vi "Test Gain.vi"(8 "error in (no error)":errorcluster, 11 "Instrument.Lockin in":refnum<class "Instrument.Lockin.lvclass">) -> (0 "error out":errorcluster, 3 "Instrument.Lockin out":refnum<class "Instrument.Lockin.lvclass">)   [LabVIEW 2019]
uses:
  src/Instrument.Lockin/Instrument.Lockin.lvclass
  <vilib>/addons/_JKI Toolkits/Caraya/classes/Assert/Assert Equal Value_Variant.vi
  <vilib>/addons/_JKI Toolkits/Caraya/classes/Test/Test.lvclass
  <vilib>/addons/_JKI Toolkits/Caraya/classes/Assert/Assert.lvclass
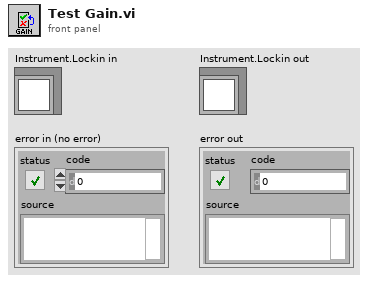
[diagram p1: front panel]
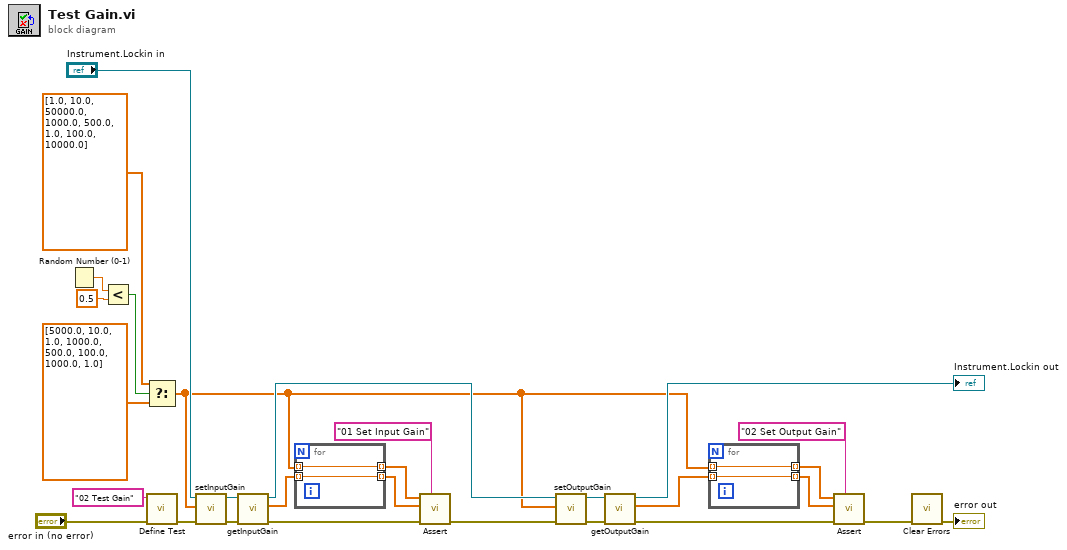
[diagram p0: block diagram]
diagram:
  n1 = Random Number (0-1)() -> (number: 0 to 1=w24:dbl)
  n2 = Less?(x=w24, y=0.5) -> (x < y?=w21:bool)
  n3 = Select(t=dbl[] [1.0, 10.0, 50000.0, 1000.0, 500.0, 1.0, 100.0, 10000.0] ("Gain"), s=w21, f=dbl[] [5000.0, 10.0, 1.0, 1000.0, 500.0, 100.0, 1000.0, 1.0] ("Gain")) -> (s? t:f=w1:dbl[])
  n4 = call <vilib>:"Define Test.vi"("error in (no error)"="error in (no error)", "Label (VI Title)"="02 Test Gain") -> ("error out"=w29:errorcluster)  [unwired: 9 in]
  n5 = call "setInputGain.vi"("error in (no error)"=w29, "InputGain"=w1, "Instrument.Lockin in"="Instrument.Lockin in") -> ("error out"=w27:errorcluster, "Instrument.Lockin out"=w26:refnum<class "Instrument.Lockin.lvclass">)  [unwired: 7 in]
  n6 = call "getInputGain.vi"("error in (no error)"=w27, "Instrument.Lockin in"=w26) -> ("error out"=w14:errorcluster, "InputGain"=w17:dbl[], "Instrument.Lockin out"=w10:refnum<class "Instrument.Lockin.lvclass">)  [unwired: 7 in]
  n7 = for {
    tunnel: [w31] -> w16 mode=indexing
    tunnel: w1 -> [w31] mode=indexing
    tunnel: [w30] -> w15 mode=indexing
    tunnel: w17 -> [w30] mode=indexing
  }
  n8 = call-poly <vilib>:"Assert.vi"("Label"="01 Set Input Gain", "error in (no error)"=w14, "Y"=w15, "X"=w16) -> ("error out"=w12:errorcluster)  [unwired: 7 in]
  n9 = call "setOutputGain.vi"("error in (no error)"=w12, "OutputGain"=w1, "Instrument.Lockin in"=w10) -> ("error out"=w11:errorcluster, "Instrument.Lockin out"=w4:refnum<class "Instrument.Lockin.lvclass">)  [unwired: 7 in]
  n10 = call "getOutputGain.vi"("error in (no error)"=w11, "Instrument.Lockin in"=w4) -> ("error out"=w6:errorcluster, "InputGain"=w5:dbl[], "Instrument.Lockin out"=→"Instrument.Lockin out":refnum<class "Instrument.Lockin.lvclass">)  [unwired: 7 in]
  n11 = for {
    tunnel: [w33] -> w7 mode=indexing
    tunnel: w1 -> [w33] mode=indexing
    tunnel: [w32] -> w8 mode=indexing
    tunnel: w5 -> [w32] mode=indexing
  }
  n12 = call-poly <vilib>:"Assert.vi"("Label"="02 Set Output Gain", "error in (no error)"=w6, "Y"=w8, "X"=w7) -> ("error out"=w2:errorcluster)  [unwired: 7 in]
  n13 = call <vilib>:"Clear Errors.vi"("error in (no error)"=w2) -> ("error out"=→"error out":errorcluster)  [unwired: 5 in, 1 out]
